vi "updateWireRule.vi"(8 "error in (no error)":errorcluster, 9 "Wire Rule":T1(ring)=enum."Recommended", 10 "terminalIndex":u32=8, 11 "PolymorphicInstance in":refnum<class "PolymorphicInstance.lvclass">) -> (0 "error out":errorcluster, 3 "PolymorphicInstance out":refnum<class "PolymorphicInstance.lvclass">)   [LabVIEW 2012, in "PolymorphicInstance.lvclass"]
uses:
  PolymorphicInstance.lvclass
  PolymorphicInstance.lvclass/PolymorphicInstance.ctl
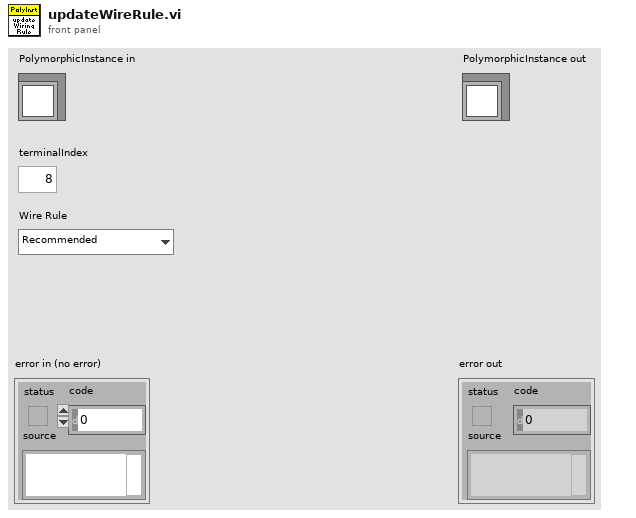
[diagram p1: front panel]
types:
  T1 = enum16{"Invalid Wire Rule", "Required", "Recommended", "Optional", "Dynamic Dispatch"}
  T2 = enum16{"Invalid Wire Rule", "Required", "Recommended", "Optional", "Dynamic Dispatch"}[]
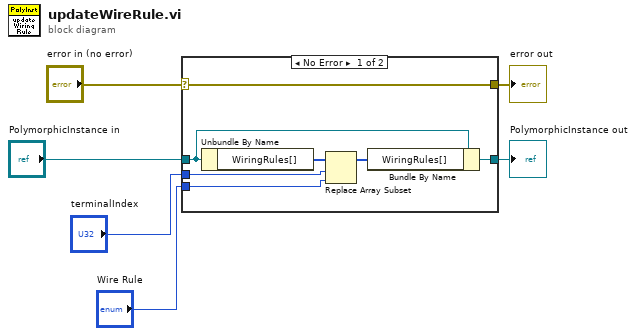
[diagram p0: block diagram]
diagram:
  n1 = case shown="No Error" "error in (no error)" {
    selector: "error in (no error)" -> [w13 w15]
    tunnel: [w13 w15] -> w5
    tunnel: [w11 w14] -> w3
    tunnel: "PolymorphicInstance in" -> [w12 w14]
    tunnel: "terminalIndex" -> [w8 _]
    tunnel: "Wire Rule" -> [w7 _]
    frame No Error {
      n2 = Unbundle By Name(w12) -> ("WiringRules[]"=w9:T2)
      n3 = Replace Array Subset(array=w9, new element=w7, index=w8) -> (w10:T2)
      n4 = Bundle By Name(cluster=w12, "WiringRules[]"=w10) -> (w11:refnum<class "PolymorphicInstance.lvclass">)
    }
    frame Error {
    }
  }
  "error out" <- w5
  "PolymorphicInstance out" <- w3
